vi "CAN Cluster Menu From Database.vi"(6 "Initialize":bool, 8 "error in":errorcluster, 9 "Default CAN Cluster Name":string, 10 "Database":T1[](array[typedef]), 11 "CAN Cluster Menu Refnum":refnum<vi>) -> (0 "error out":errorcluster)   [LabVIEW 2020, in "Communication Bus Template System Explorer.lvlib" / "Implementation.lvlib"]
uses:
  Implementation.lvlib
  Types/CAN Cluster.ctl
  Types/Database.ctl
  Types/Frame.ctl
  Types/Signal.ctl
  Types/ECU.ctl
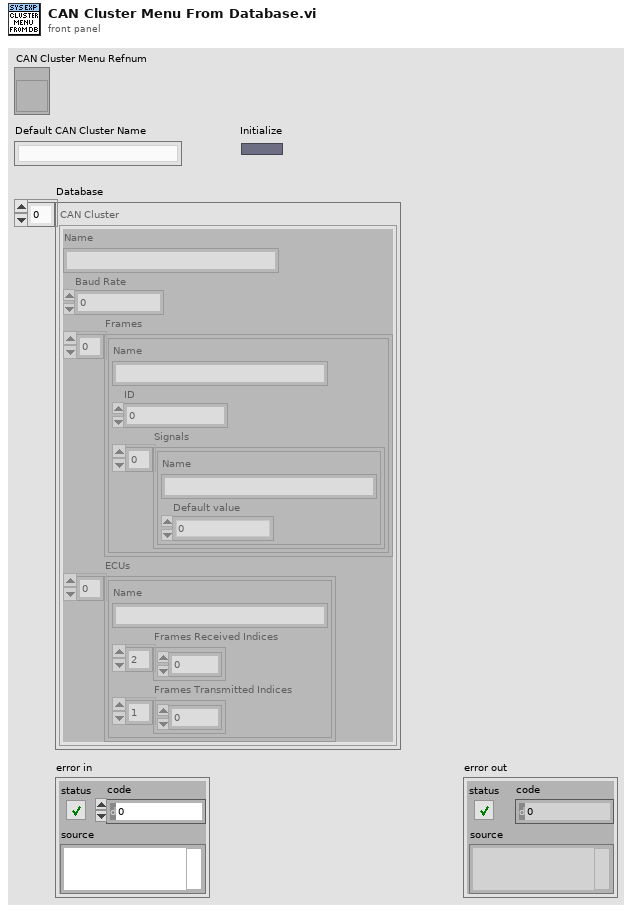
[diagram p1: front panel]
types:
  T1 = typedef "Communication Bus Template System Explorer.lvlib/Implementation.lvlib/Database.ctl" = cluster{"Name":string, "Baud Rate":u64, "Frames":T2[], "ECUs":T4[]}
  T2 = typedef "Communication Bus Template System Explorer.lvlib/Implementation.lvlib/Frame.ctl" = cluster{"Name":string, "ID":u32, "Signals":T3[]}
  T3 = typedef "Communication Bus Template System Explorer.lvlib/Implementation.lvlib/Signal.ctl" = cluster{"Name":string, "Default value":dbl}
  T4 = typedef "Communication Bus Template System Explorer.lvlib/Implementation.lvlib/ECU.ctl" = cluster{"Name":string, "Frames Received Indices":u32[], "Frames Transmitted Indices":u32[]}
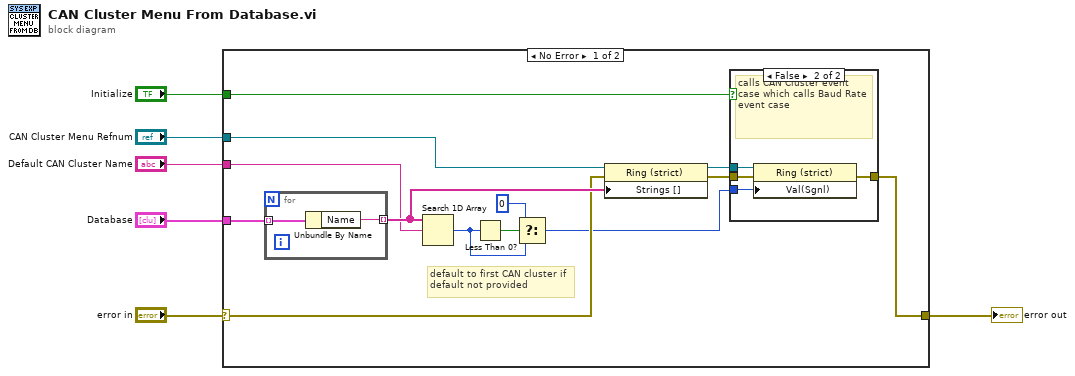
[diagram p0: block diagram]
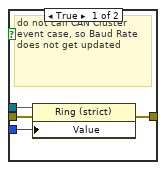
[diagram p2: hidden frame]
diagram:
  n1 = case shown="No Error" "error in" {
    selector: "error in" -> [w13 w30]
    tunnel: "CAN Cluster Menu Refnum" -> [w18 _]
    tunnel: "Database" -> [w17 _]
    tunnel: "Default CAN Cluster Name" -> [w16 _]
    tunnel: [w10 w30] -> w2
    tunnel: "Initialize" -> [w7 _]
    frame No Error {
      # "default to first CAN cluster if default not provided"
      n2 = for {
        tunnel: w17 -> [w29] mode=indexing
        tunnel: [w28] -> w19 mode=indexing
        n3 = Unbundle By Name(w29) -> ("Name"=w28:string)
      }
      n4 = Search 1D Array(1D array=w19, element=w16) -> (index of element=w15:i32)  [unwired: 1 in]
      n5 = Less Than 0?(x=w15) -> (x < 0?=w8:bool)
      n6 = Select(t=0, s=w8, f=w15) -> (s? t:f=w9:i32)
      n7 = property on="Property Node" class="Ring (strict)"(reference=w18, error in=w13, "Strings []"=w19) -> (reference out=w12:refnum<vi>, error out=w11:errorcluster)
      n8 = case shown="False" w7 {
        tunnel: w12 -> [w23 w27]
        tunnel: w11 -> [w22 w26]
        tunnel: [w21 w25] -> w10
        tunnel: w9 -> [w20 w24]
        frame True {
          # "do not call CAN Cluster event case, so Baud Rate does not get updated"
          n9 = property on="Property Node" class="Ring (strict)"(reference=w23, error in=w22, "Value"=w20) -> (error out=w21:errorcluster)  [unwired: 1 out]
        }
        frame False {
          # "calls CAN Cluster event case which calls Baud Rate event case"
          n10 = property on="Property Node" class="Ring (strict)"(reference=w27, error in=w26, "Val(Sgnl)"=w24) -> (error out=w25:errorcluster)  [unwired: 1 out]
        }
      }
    }
    frame Error {
    }
  }
  "error out" <- w2
